vi "Bundle.vi"(7 "Restore Range if Changed?(T)":bool=TRUE, 8 "error in (no error)":errorcluster, 9 "Max Time(-1ms)":i32=-1, 10 "Measurements to Acquire(1)":i32=1, 11 "DMM Immediate Measure Msg in":refnum<class "DMM Immediate Measure Msg.lvclass">) -> (0 "error out":errorcluster, 3 "DMM Immediate Measure Msg out":refnum<class "DMM Immediate Measure Msg.lvclass">)   [LabVIEW 2020, in "DMM Msg.lvlib" / "DMM Immediate Measure Msg.lvclass"]
doc: "Populate the message."
uses:
  DMM Immediate Measure Msg.lvclass
  DMM Immediate Measure Msg.lvclass/DMM Immediate Measure Msg.ctl
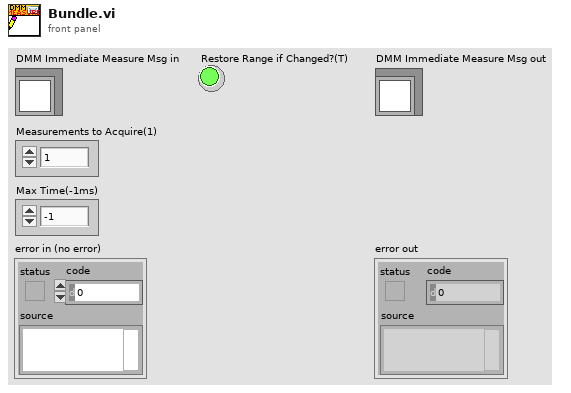
[diagram p1: front panel]
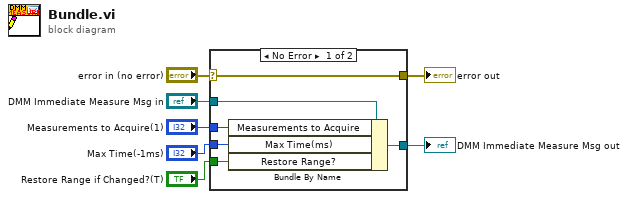
[diagram p0: block diagram]
diagram:
  n1 = case shown="No Error" "error in (no error)" {
    selector: "error in (no error)" -> [w13 w14]
    tunnel: [w13 w14] -> w6
    tunnel: [w11 w15] -> w4
    tunnel: "DMM Immediate Measure Msg in" -> [w12 w15]
    tunnel: "Measurements to Acquire(1)" -> [w10 _]
    tunnel: "Max Time(-1ms)" -> [w9 _]
    tunnel: "Restore Range if Changed?(T)" -> [w8 _]
    frame No Error {
      n2 = Bundle By Name(cluster=w12, "Measurements to Acquire"=w10, "Max Time(ms)"=w9, "Restore Range?"=w8) -> (w11:refnum<class "DMM Immediate Measure Msg.lvclass">)
    }
    frame Error {
    }
  }
  "error out" <- w6
  "DMM Immediate Measure Msg out" <- w4
